vi "GetPumpHandle.vi"(0 "object in":refnum<class "CetoniPump.lvclass">, 2 "index":i32, 5 "error in (no error)":errorcluster) -> (14 "object out":refnum<class "CetoniPump.lvclass">, 15 "Pump handle":i64, 19 "error out":errorcluster)   [LabVIEW 2023, in "CetoniPump.lvclass"]
uses:
  CetoniPump.lvclass
  CetoniPump.lvclass/CetoniPump.ctl
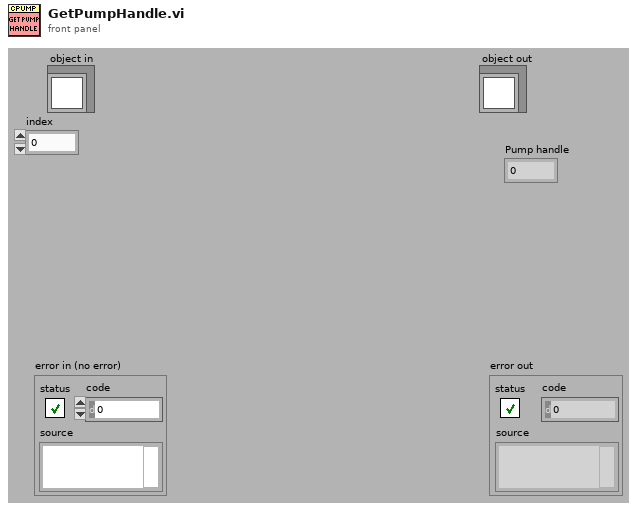
[diagram p1: front panel]
types:
  T1 = cluster{"Pump Handle":i64, "Pump Name":string, "Maximum Volume":dbl, "Maximum Flow Rate":dbl, "Flow Rate":dbl, "Target Level":dbl, "Valve Handle":i64, "Has Valve?":bool, "Actual valve position":i32}[]
  T2 = cluster{"Pump Handle":i64, "Pump Name":string, "Maximum Volume":dbl, "Maximum Flow Rate":dbl, "Flow Rate":dbl, "Target Level":dbl, "Valve Handle":i64, "Has Valve?":bool, "Actual valve position":i32}
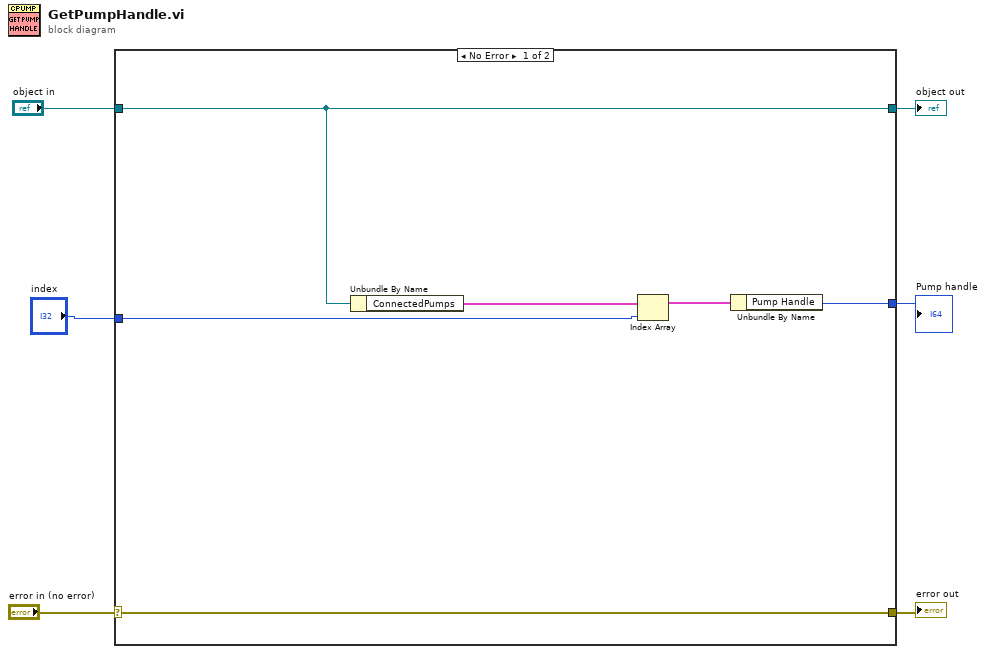
[diagram p0: block diagram]
diagram:
  n1 = case shown="No Error" "error in (no error)" {
    selector: "error in (no error)" -> [w11 w14]
    tunnel: [w11 w14] -> w5
    tunnel: [w10 w13] -> w3
    tunnel: "object in" -> [w10 w13]
    tunnel: [w7 _] -> w2
    tunnel: "index" -> [w8 _]
    frame No Error {
      n2 = Unbundle By Name(w10) -> ("ConnectedPumps"=w12:T1)
      n3 = Index Array(array=w12, index=w8) -> (element=w9:T2)
      n4 = Unbundle By Name(w9) -> ("Pump Handle"=w7:i64)
    }
    frame Error {
    }
  }
  "error out" <- w5
  "object out" <- w3
  "Pump handle" <- w2
